vi "3458A Self Calibrate Virtual Channels.vi"(8 "error in":errorcluster, 11 "digitizer session in":T1 {"channels"."Range [Vpk]" min=0.0}) -> (0 "error":errorcluster, 3 "digitizer session out":T1 {"channels"."Range [Vpk]" min=0.0})   [LabVIEW 2018, in "3458A Virtual Digitizer.lvlib"]
doc: "This VI will allow user to initiate AUTOCAL function on all virtual channels. It will perform DCV calibartion and when the DSDC or DSAC mode is selected it will also perform ACV calibration."
uses:
  3458A Virtual Digitizer.lvlib
  3458A Digitizer Session.ctl
  3458A Virtual Channel Config.ctl
  Counter/Counter Session.ctl
  Counter/Counter Type.ctl
  AWG/AWG Session.ctl
  AWG/AWG Type.ctl
  3458A Sync Mode.ctl
  3458A Idn Mode.ctl
  3458A Digitizing Low Levels/Configure/Sampling Mode.ctl
  3458A Digitizing Process Options.ctl
  3458A Data Packet.ctl
  3458A Aux Record Data.ctl
  3458A Digitizing Low Levels/Configure/Level Setup.ctl
  3458A Digitizing Low Levels/Configure/First Sample Trigger.ctl
  3458A Aperture Selection Mode.ctl
  3458A Digitizing Low Levels/Action-Status/AutoCal Mode.ctl
  3458A Digitizing Low Levels/3458A Digitizing Low Levels.lvlib
  3458A Basic Driver/3458A Basic Driver.lvlib
  Counter/Counter.lvlib
  AWG/AWG.lvlib
panel:
  in  "btn abort":bool
  in  "btn exit":bool
  in  "btn start":bool
  out "Status":string
  out "state":i32
  # "1) Disconnect everything from inputs of the DMMs. \n2) Press start to start AUTOCAL.\n3) When done, leave by EXIT.\n4) If it goes wrong, use ABORT to terminate."
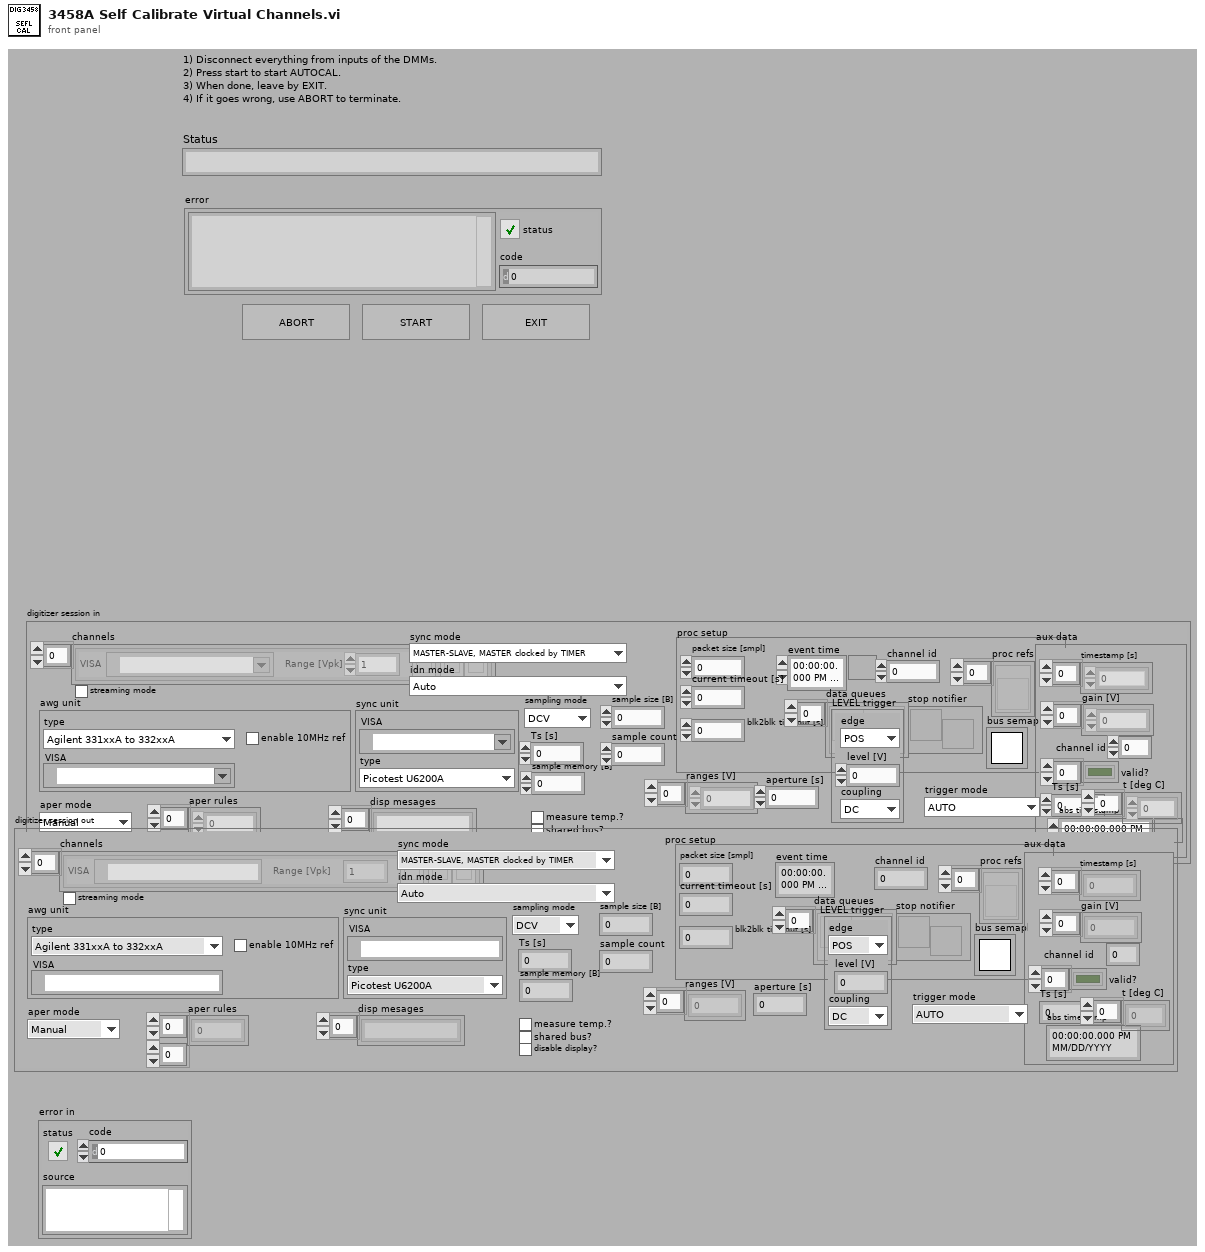
[diagram p1: front panel]
types:
  T1 = typedef "3458A Virtual Digitizer.lvlib/3458A Digitizer Session.ctl" = cluster{"channels":T2[], "sync unit":T3, "awg unit":T5, "sync mode":T7, "streaming mode":bool, "idn mode":T8, "sampling mode":T9, "Ts [s]":dbl, "sample memory [B]":i32, "proc setup":T10, "sample size [B]":i32, "sample count":i32, "aux data":T12, "ranges [V]":dbl[], "aperture [s]":dbl, "LEVEL trigger":T13, "trigger mode":T14, "measure temp.?":bool, "disp mesages":string[], "shared bus?":bool, "disable display?":bool, "aper mode":T15, "aper rules":dbl[][]}
  T2 = typedef "3458A Virtual Digitizer.lvlib/3458A Virtual Channel Config.ctl" = cluster{"VISA":refnum<visa-resource-name>, "Range [Vpk]":dbl, "btn clr":bool, "btn up":bool, "btn down":bool}
  T3 = typedef "Counter.lvlib/Counter Session.ctl" = cluster{"VISA":refnum<visa-resource-name>, "type":T4}
  T4 = typedef "Counter.lvlib/Counter Type.ctl" = enum16{"Picotest U6200A", "dummy"}
  T5 = typedef "AWG.lvlib/AWG Session.ctl" = cluster{"type":T6, "VISA":refnum<visa-resource-name>, "enable 10MHz ref":bool}
  T6 = typedef "AWG.lvlib/AWG Type.ctl" = enum16{"Agilent 331xxA to 332xxA", "Agilent 335xxA to 336xxA", "Tektronix AFG3101C", "dummy"}
  T7 = typedef "3458A Virtual Digitizer.lvlib/3458A Sync Mode.ctl" = enum16{"MASTER-SLAVE, MASTER clocked by TIMER", "MASTER-SLAVE, MASTER clocked by AWG", "ALL clocked by AWG", "MASTER-SLAVE, ALL clocked by TIMER", "ALL clocked by AWG with DFLL"}
  T8 = typedef "3458A Virtual Digitizer.lvlib/3458A Idn Mode.ctl" = enum16{"Auto", "Sequential (chn A, chn B, ...)", "From calibration string"}
  T9 = typedef "3458A Virtual Digitizer.lvlib/3458A Digitizing Low Levels.lvlib/Sampling Mode.ctl" = enum16{"DCV", "DSDC", "DSAC"}
  T10 = typedef "3458A Virtual Digitizer.lvlib/3458A Digitizing Process Options.ctl" = cluster{"channel id":i32, "packet size [smpl]":i32, "current timeout [s]":dbl, "blk2blk timeout [s]":dbl, "event time":timestamp, "stop notifier":refnum<notifier>, "data queues":refnum<queue>[], "proc refs":refnum<vi>[], "bus semaphore":T11}
  T11 = typedef "Semaphore RefNum" = refnum<k1>
  T12 = typedef "3458A Virtual Digitizer.lvlib/3458A Aux Record Data.ctl" = cluster{"channel id":i32, "valid?":bool[], "gain [V]":dbl[], "timestamp [s]":dbl[], "Ts [s]":dbl, "abs timestamp":timestamp, "t [deg C]":dbl[]}
  T13 = typedef "3458A Virtual Digitizer.lvlib/3458A Digitizing Low Levels.lvlib/Level Setup.ctl" = cluster{"edge":enum16{"POS", "NEG"}, "level [V]":dbl, "coupling":enum16{"DC", "AC"}}
  T14 = typedef "3458A Virtual Digitizer.lvlib/3458A Digitizing Low Levels.lvlib/First Sample Trigger.ctl" = enum16{"AUTO", "EXT", "SYN", "SGL", "HOLD", "LEVEL"}
  T15 = typedef "3458A Virtual Digitizer.lvlib/3458A Aperture Selection Mode.ctl" = enum16{"Manual", "Maximum", "Table"}
  T16 = typedef "3458A Virtual Digitizer.lvlib/3458A Digitizing Low Levels.lvlib/AutoCal Mode.ctl" = enum16{"ALL", "DCV", "AC", "OHMS"}
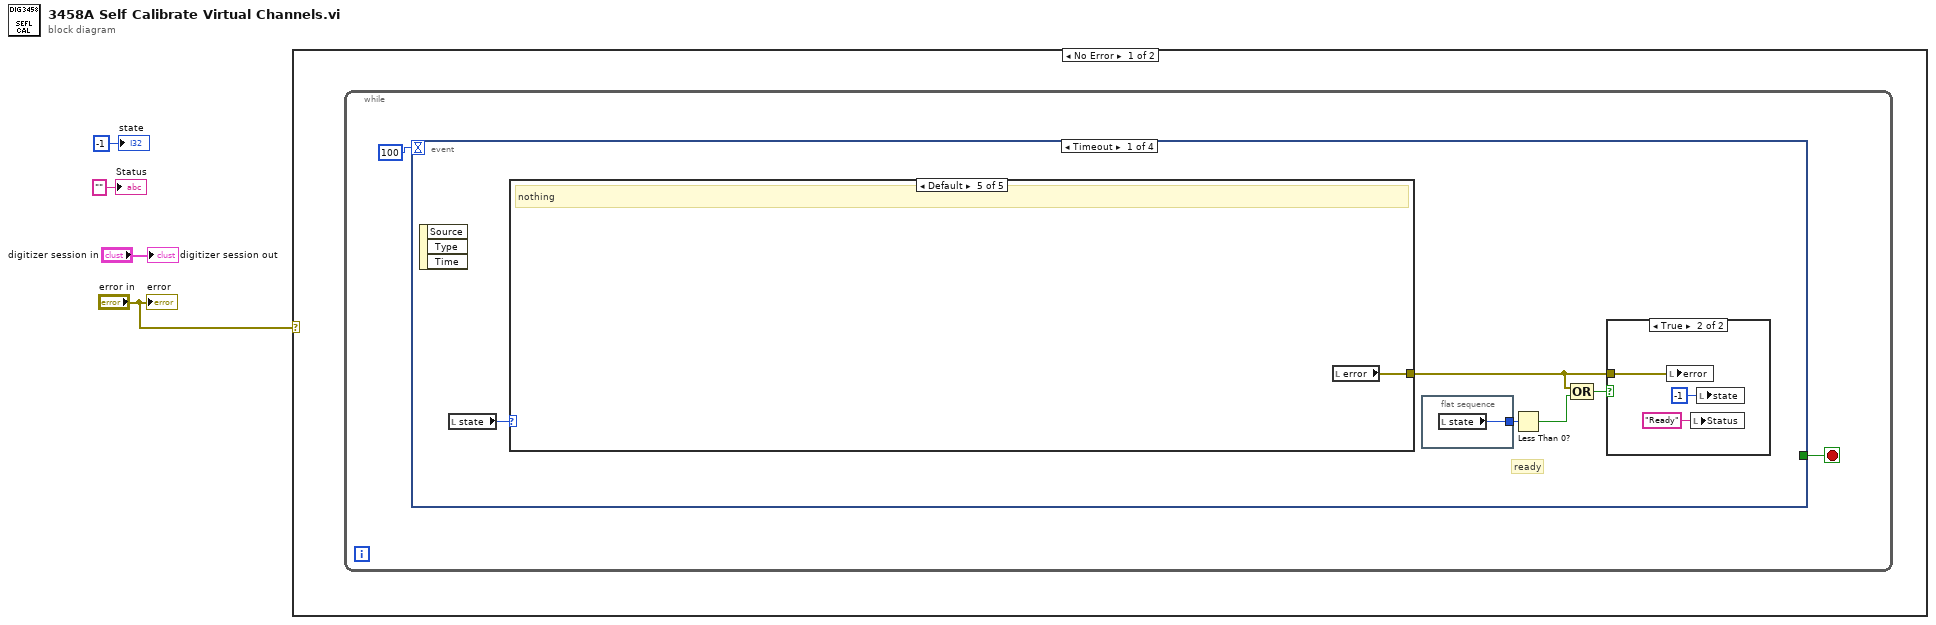
[diagram p0: block diagram]
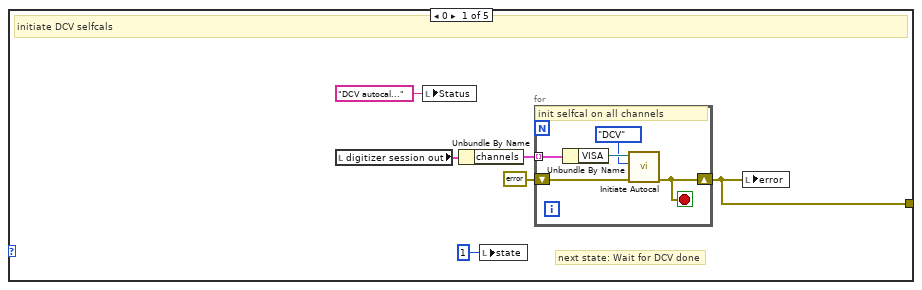
[diagram p3: hidden frame]
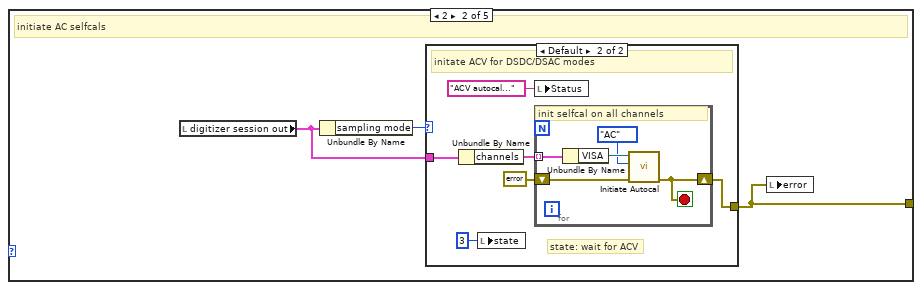
[diagram p4: hidden frame]
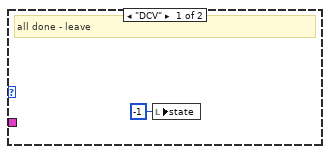
[diagram p5: hidden frame]
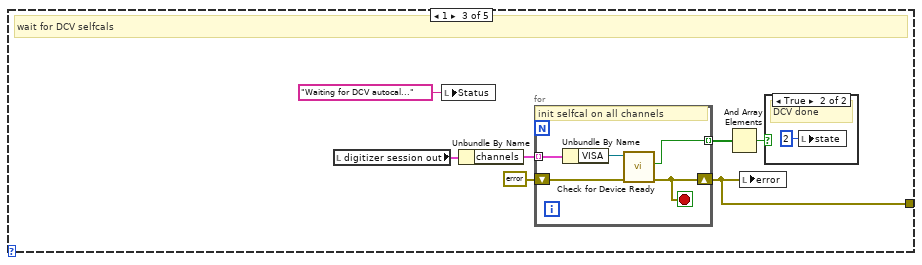
[diagram p6: hidden frame]
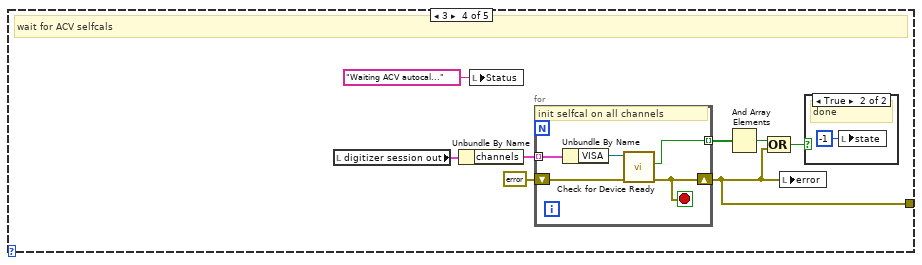
[diagram p8: hidden frame]
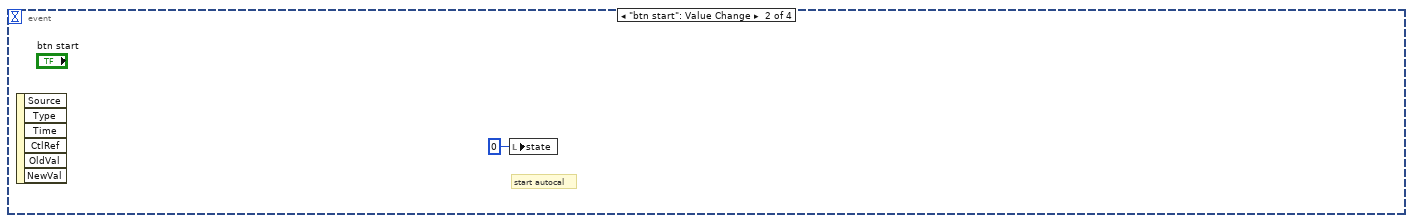
[diagram p10: hidden frame]
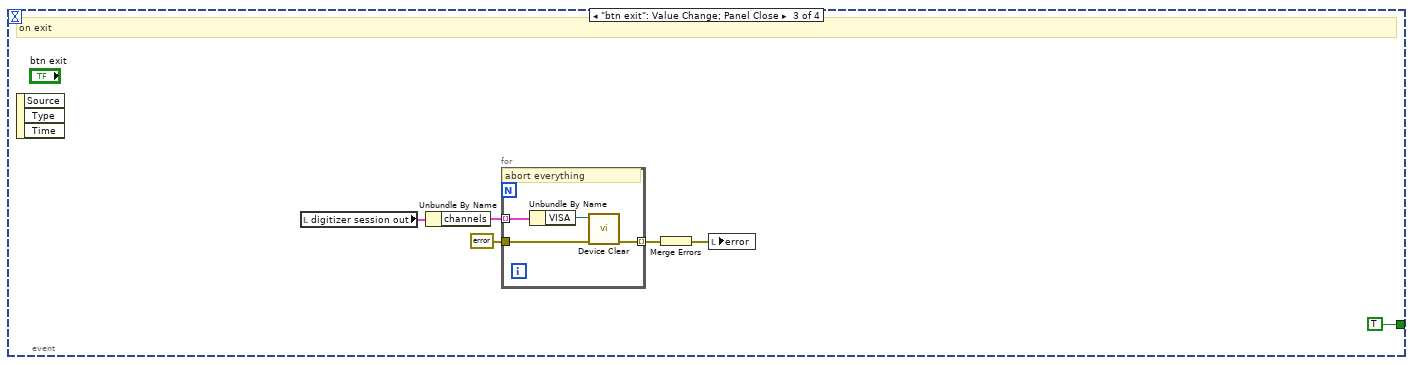
[diagram p11: hidden frame]
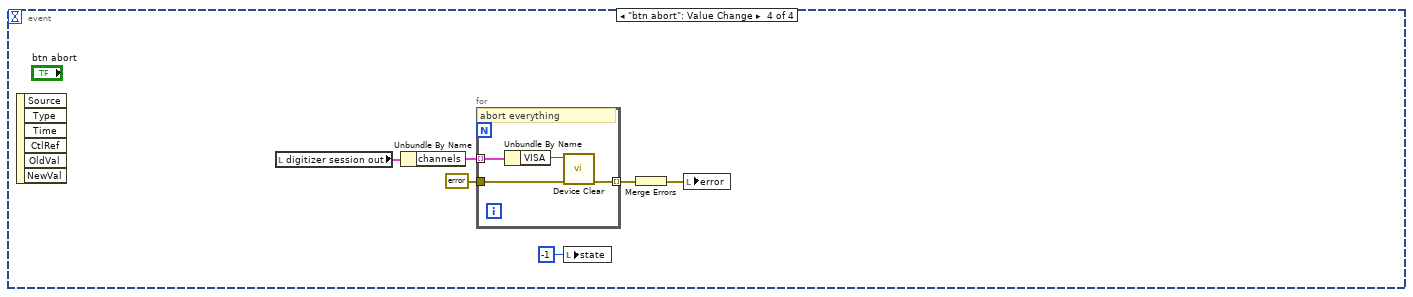
[diagram p12: hidden frame]
diagram:
  n1 = case shown="No Error" "error in" {
    frame No Error {
      n2 = while {
        stop <- w5 stop-if-true
        n3 = event shown="[0] Timeout" {
          selector: _ -> [_ _ _ _]
          dyn-events: _ -> [_ _ _ _]
          timeout: 100 -> [_ _ _ _]
          tunnel: [_ _ TRUE _] -> w5
          event Timeout {
            # "ready"
            n4 = event-data() -> ()  [unwired: 1 in, 3 out]
            n5 = local read "state"() -> (w11:i32)
            n6 = case shown="Default" w11 {
              tunnel: [w16 w29 w46 w55 w69] -> w9
              frame 0 {
                # "next state: Wait for DCV done"
                # "initiate DCV selfcals"
                n7 = local read "digitizer session out"() -> (w18:T1)
                n8 = local write "Status"("DCV autocal..." ("Status")) -> ()
                n9 = Unbundle By Name(w18) -> ("channels"=w21:T2[])
                n10 = local write "state"(1) -> ()
                n11 = for {
                  tunnel: w21 -> [w24] mode=indexing
                  shift-right: [w23] -> w16
                  shift-left: errorcluster {"status"=FALSE, "code"=0, "source"=""} ("error out") -> [w26]
                  stop <- w23 stop-if-true
                  # "init selfcal on all channels"
                  n12 = Unbundle By Name(w24) -> ("VISA"=w25:refnum<visa-resource-name>)
                  n13 = call "Initiate Autocal.vi"("error in"=w26, "mode (ALL)"=AutoCal_Mode."DCV", "VISA resource in"=w25) -> ("error out"=w23:errorcluster)  [unwired: 7 in, 1 out]
                }
                n14 = local write "error"(w16) -> ()
              }
              frame 2 {
                # "initiate AC selfcals"
                n15 = local read "digitizer session out"() -> (w28:T1)
                n16 = Unbundle By Name(w28) -> ("sampling mode"=w27:T9)
                n17 = case shown="Default" w27 {
                  tunnel: [_ w34] -> w29
                  tunnel: w28 -> [_ w33]
                  frame "DCV" {
                    # "all done - leave"
                    n18 = local write "state"(-1) -> ()
                  }
                  frame Default {
                    # "state: wait for ACV"
                    # "initate ACV for DSDC/DSAC modes"
                    n19 = Unbundle By Name(w33) -> ("channels"=w36:T2[])
                    n20 = local write "state"(3 ("state")) -> ()
                    n21 = local write "Status"("ACV autocal..." ("Status")) -> ()
                    n22 = for {
                      tunnel: w36 -> [w39] mode=indexing
                      shift-right: [w38] -> w34
                      shift-left: errorcluster {"status"=FALSE, "code"=0, "source"=""} ("error out") -> [w41]
                      stop <- w38 stop-if-true
                      # "init selfcal on all channels"
                      n23 = Unbundle By Name(w39) -> ("VISA"=w40:refnum<visa-resource-name>)
                      n24 = call "Initiate Autocal.vi"("error in"=w41, "mode (ALL)"=AutoCal_Mode."AC", "VISA resource in"=w40) -> ("error out"=w38:errorcluster)  [unwired: 7 in, 1 out]
                    }
                  }
                }
                n25 = local write "error"(w29) -> ()
              }
              frame 1 {
                # "wait for DCV selfcals"
                n26 = local read "digitizer session out"() -> (w43:T1)
                n27 = local write "Status"("Waiting for DCV autocal..." ("Status")) -> ()
                n28 = Unbundle By Name(w43) -> ("channels"=w48:T2[])
                n29 = for {
                  tunnel: w48 -> [w52] mode=indexing
                  shift-right: [w51] -> w46
                  shift-left: errorcluster {"status"=FALSE, "code"=0, "source"=""} ("error out") -> [w54]
                  tunnel: [w50] -> w45 mode=indexing
                  stop <- w51 stop-if-true
                  # "init selfcal on all channels"
                  n30 = Unbundle By Name(w52) -> ("VISA"=w53:refnum<visa-resource-name>)
                  n31 = call "Check for Device Ready.vi"("error in"=w54, "VISA resource in"=w53) -> ("error out"=w51:errorcluster, "device ready?"=w50:bool)  [unwired: 7 in, 1 out]
                }
                n32 = And Array Elements(Boolean array=w45) -> (logical AND=w44:bool)
                n33 = local write "error"(w46) -> ()
                n34 = case shown="True" w44 {
                  frame False {
                  }
                  frame True {
                    # "DCV done"
                    n35 = local write "state"(2 ("state")) -> ()
                  }
                }
              }
              frame 3 {
                # "wait for ACV selfcals"
                n36 = local read "digitizer session out"() -> (w59:T1)
                n37 = Unbundle By Name(w59) -> ("channels"=w62:T2[])
                n38 = local write "Status"("Waiting ACV autocal..." ("Status")) -> ()
                n39 = for {
                  tunnel: w62 -> [w66] mode=indexing
                  shift-right: [w65] -> w55
                  shift-left: errorcluster {"status"=FALSE, "code"=0, "source"=""} ("error out") -> [w68]
                  tunnel: [w64] -> w60 mode=indexing
                  stop <- w65 stop-if-true
                  # "init selfcal on all channels"
                  n40 = Unbundle By Name(w66) -> ("VISA"=w67:refnum<visa-resource-name>)
                  n41 = call "Check for Device Ready.vi"("error in"=w68, "VISA resource in"=w67) -> ("error out"=w65:errorcluster, "device ready?"=w64:bool)  [unwired: 7 in, 1 out]
                }
                n42 = And Array Elements(Boolean array=w60) -> (logical AND=w57:bool)
                n43 = Compound Arithmetic op=OR(w57, w55) -> (w56:bool)
                n44 = local write "error"(w55) -> ()
                n45 = case shown="True" w56 {
                  frame False {
                  }
                  frame True {
                    # "done"
                    n46 = local write "state"(-1 ("state")) -> ()
                  }
                }
              }
              frame Default {
                # "nothing"
                n47 = local read "error"() -> (w69:errorcluster)
              }
            }
            n48 = flat-sequence {
              tunnel: [w15] -> w10
              frame #0 {
                n49 = local read "state"() -> (w15:i32)
              }
            }
            n50 = Less Than 0?(x=w10) -> (x < 0?=w8:bool)
            n51 = Compound Arithmetic op=OR(w9, w8) -> (w7:bool)
            n52 = case shown="True" w7 {
              tunnel: w9 -> [_ w13]
              frame False {
              }
              frame True {
                n53 = local write "error"(w13) -> ()
                n54 = local write "Status"("Ready" ("Status")) -> ()
                n55 = local write "state"(-1 ("state")) -> ()
              }
            }
          }
          event "btn start": Value Change {
            # "start autocal"
            n56 = event-data() -> ()  [unwired: 1 in, 6 out]
            n57 = local write "state"(0 ("state")) -> ()
          }
          event "btn exit": Value Change; Panel Close {
            # "on exit"
            n58 = event-data() -> ()  [unwired: 1 in, 3 out]
            n59 = local read "digitizer session out"() -> (w74:T1)
            n60 = Unbundle By Name(w74) -> ("channels"=w76:T2[])
            n61 = for {
              tunnel: w76 -> [w80] mode=indexing
              tunnel: errorcluster {"status"=FALSE, "code"=0, "source"=""} ("error out") -> [w79]
              tunnel: [w77] -> w73 mode=indexing
              # "abort everything"
              n62 = Unbundle By Name(w80) -> ("VISA"=w78:refnum<visa-resource-name>)
              n63 = call "Device Clear.vi"("error in(no error)"=w79, "VISA Resource Name"=w78) -> ("error out"=w77:errorcluster)  [unwired: 8 in, 1 out]
            }
            n64 = Merge Errors(w73) -> (w72:errorcluster)
            n65 = local write "error"(w72) -> ()
          }
          event "btn abort": Value Change {
            n66 = event-data() -> ()  [unwired: 1 in, 6 out]
            n67 = local read "digitizer session out"() -> (w84:T1)
            n68 = Unbundle By Name(w84) -> ("channels"=w86:T2[])
            n69 = for {
              tunnel: w86 -> [w90] mode=indexing
              tunnel: errorcluster {"status"=FALSE, "code"=0, "source"=""} ("error out") -> [w89]
              tunnel: [w87] -> w83 mode=indexing
              # "abort everything"
              n70 = Unbundle By Name(w90) -> ("VISA"=w88:refnum<visa-resource-name>)
              n71 = call "Device Clear.vi"("error in(no error)"=w89, "VISA Resource Name"=w88) -> ("error out"=w87:errorcluster)  [unwired: 8 in, 1 out]
            }
            n72 = local write "state"(-1 ("state")) -> ()
            n73 = Merge Errors(w83) -> (w82:errorcluster)
            n74 = local write "error"(w82) -> ()
          }
        }
      }
    }
    frame Error {
    }
  }
  "digitizer session out" <- "digitizer session in"
  "error" <- "error in"
  "state" <- -1 ("state")
  "Status" <- "" ("Status")
